vi "Check CS Lines vs Devices.vi"(8 "error in":errorcluster, 11 "Bus Info":T1[](array[typedef])) -> (0 "error out":errorcluster)   [LabVIEW 2014, in "SPI Engine Scripting.lvlib"]
doc: "Checks if there is one chip select line selected per device. If not, it throws a custom error."
uses:
  SPI Engine Scripting.lvlib
  State Machine/Controls/Bus Information.ctl
  State Machine/Controls/Device Information.ctl
  <vilib>/LabVIEW Icon API/API_Text.ctl
  State Machine/Controls/Pin Information.ctl
  <vilib>/LabVIEW Icon API/LabVIEW Icon API.lvlib
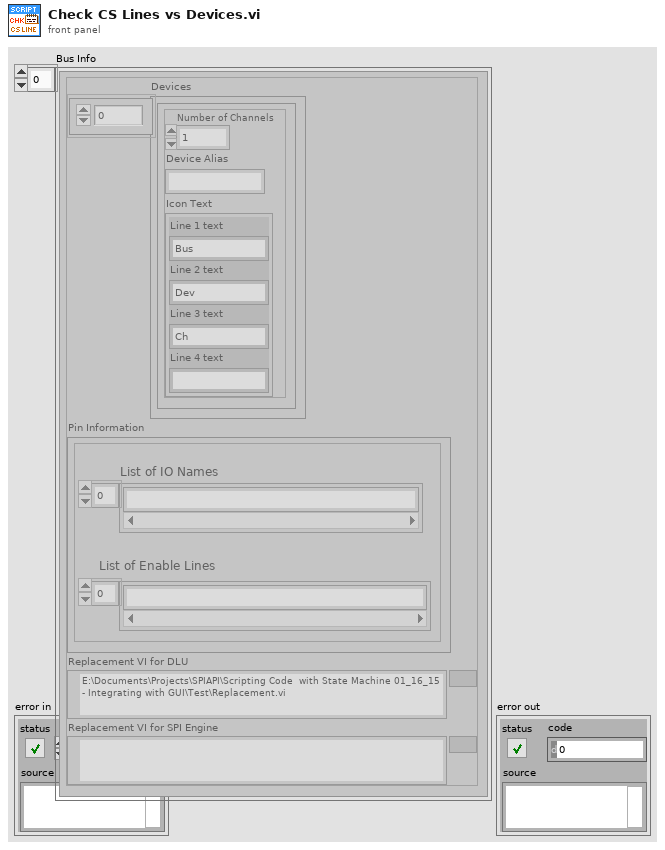
[diagram p1: front panel]
types:
  T1 = typedef "SPI Engine Scripting.lvlib/Bus Information.ctl" = cluster{"Devices":T2[], "Pin Information":T4, "Replacement VI for DLU":path, "Replacement VI for SPI Engine":path}
  T2 = typedef "Device Information.ctl" = cluster{"Number of Channels":i32, "Device Alias":string, "Icon Text":T3}
  T3 = typedef "LabVIEW Icon API.lvlib/API_Text.ctl" = cluster{"Line 1 text":string, "Line 2 text":string, "Line 3 text":string, "Line 4 text":string}
  T4 = typedef "Pin Information.ctl" = cluster{"List of IO Names":string[], "List of Enable Lines":string[]}
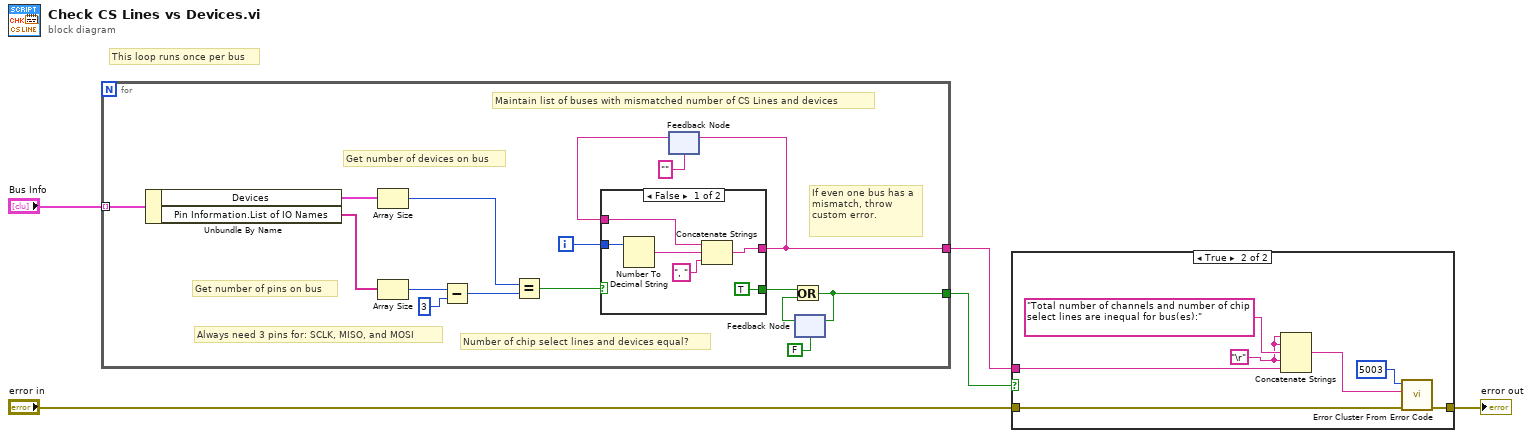
[diagram p0: block diagram]
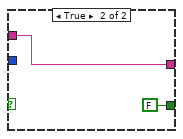
[diagram p3: hidden frame]
diagram:
  # "This loop runs once per bus"
  n1 = for {
    tunnel: "Bus Info" -> [w21] mode=indexing
    tunnel: [w12] -> w4
    tunnel: [w8] -> w5
    i -> [w16]
    # "Number of chip select lines and devices equal?"
    # "Get number of pins on bus"
    # "Get number of devices on bus"
    # "If even one bus has a mismatch, throw custom error."
    # "Maintain list of buses with mismatched number of CS Lines and devices"
    # "Always need 3 pins for: SCLK, MISO, and MOSI"
    n2 = Unbundle By Name(w21) -> ("Devices"=w7:T2[], "Pin Information.List of IO Names"=w20:string[])
    n3 = Array Size(array=w7) -> (size(s)=w6:i32)
    n4 = Array Size(array=w20) -> (size(s)=w19:i32)
    n5 = Subtract(x=w19, y=3) -> (x-y=w17:i32)
    n6 = Equal?(x=w6, y=w17) -> (x = y?=w15:bool)
    n7 = feedback #1("") -> (w14:string)
    n8 = case shown="False" w15 {
      tunnel: w16 -> [w27 _]
      tunnel: [w26 w29] -> w12
      tunnel: w14 -> [w24 w29]
      tunnel: [TRUE FALSE] -> w11
      frame False {
        n9 = Number To Decimal String(number=w27) -> (decimal integer string=w25:string)  [unwired: 1 in]
        n10 = Concatenate Strings(w24, w25, ", " ("string")) -> (w26:string)
      }
      frame True {
      }
    }
    n11 = feedback-in #1(w12) -> ()
    n12 = feedback #2(FALSE) -> (w9:bool)
    n13 = Or(x=w11, y=w9) -> (x .or. y?=w8:bool)
    n14 = feedback-in #2(w8) -> ()
  }
  n15 = case shown="True" w5 {
    tunnel: "error in" -> [w30 w37]
    tunnel: [w30 w35] -> w3
    tunnel: w4 -> [_ w32]
    frame False {
    }
    frame True {
      w31 = "\r"
      n16 = Concatenate Strings(w31, w31, "Total number of channels and number of chip select lines are inequal for bus(es):" ("error message (\"\")"), w31, w32) -> (w33:string)
      n17 = call <vilib>:"Error Cluster From Error Code.vi"("error in (no error)"=w37, "error message (\"\")"=w33, "error code (0)"=5003) -> ("error out"=w35:errorcluster)  [unwired: 6 in]
    }
  }
  "error out" <- w3
